vi "Is Sub-Path.vi"(9 "File Path 2":path, 11 "File Path":path) -> (0 "Relative File Path 2":path, 2 "File Path 2 a Sub-Path?":bool)   [LabVIEW 2010]
doc: "<B>Name:</B>\n Is Sub-Path.vi\n<B>References:</B>\n\n<B>Function Description:</B>\nThis VI returns TRUE if File Path 2 is a sub-path of File Path. It also returns the relative path from File Path to File Path 2.\n\nNote that a TRUE does not guarantee that the file path(s) exist or are valid.\n<B>Inputs:</B>\nFile path: Input path\nFile path 2: Input path for determining if if it is a sub-path of File Path.\n<B>Outputs:</B>\nFile Path 2 is a Sub Path?: Boolean result\nRelative file path 2: Relative path from File Path to File Path 2\n<B>Globals:</B>\n\n<B>TestStand Variables:</B>\n\n<B>User Guide:</B>\n\n<B>Control Usage Rules:</B>\n\n<B>VI Interaction:</B>\n\n<B>Occurences:</B>\n\n<B>Devices:</B>\n\n<B>Files:</B>\n\n<B>System Calls:</B>\n\n<B>Keywords:</B>\n\n<B>Initial Developer: Date:</B>\nMJShultz\n\nCurrent Revision: 26\nVSS Version: 3\nCopyright 2002 VI Engineering, Inc."
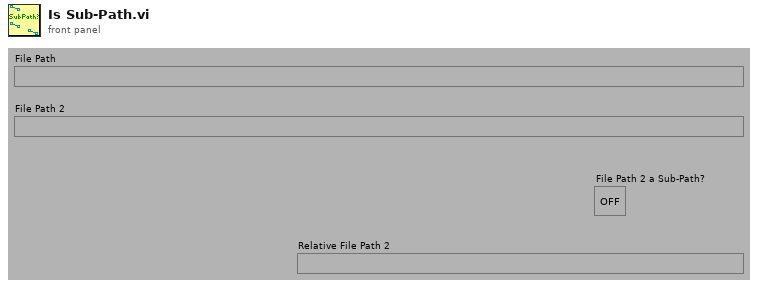
[diagram p1: front panel]
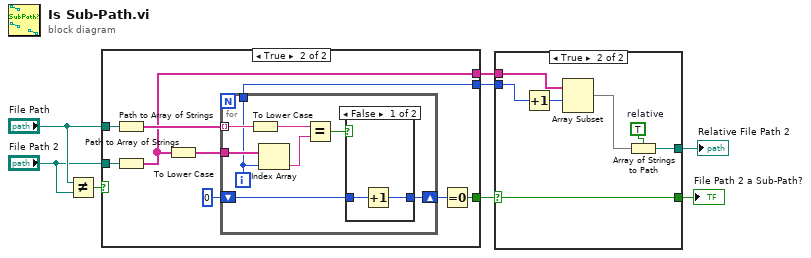
[diagram p0: block diagram]
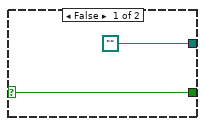
[diagram p2: hidden frame]
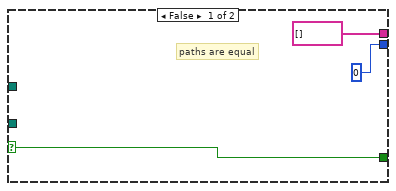
[diagram p3: hidden frame]
diagram:
  n1 = Not Equal?(x="File Path", y="File Path 2") -> (x != y?=w6:bool)
  n2 = case shown="True" w6 {
    selector: w6 -> [w11 _]
    tunnel: [w11 w17] -> w5
    tunnel: "File Path" -> [_ w16]
    tunnel: "File Path 2" -> [_ w15]
    tunnel: [0 w14] -> w3
    tunnel: [string[] [] ("array of strings") w13] -> w2
    frame False {
      # "paths are equal"
    }
    frame True {
      n3 = Path to Array of Strings(0:w16) -> (2:w20:string[])  [unwired: 1 out]
      n4 = Path to Array of Strings(0:w15) -> (2:w13:string[])  [unwired: 1 out]
      n5 = To Lower Case(string=w13) -> (all lower case string=w12:string[])
      n6 = for {
        tunnel: w20 -> [w26] mode=indexing
        tunnel: w12 -> [w28]
        shift-right: [w25] -> w18
        shift-left: 0 -> [w23]
        tunnel: [w22] -> w14
        i -> [w22]
        n7 = To Lower Case(string=w26) -> (all lower case string=w21:string)
        n8 = Index Array(array=w28, index=w22) -> (element=w27:string)
        n9 = Equal?(x=w21, y=w27) -> (x = y?=w24:bool)
        n10 = case shown="False" w24 {
          tunnel: [w29 w31] -> w25
          tunnel: w23 -> [w30 w31]
          frame False {
            n11 = Increment(x=w30) -> (x+1=w29:i32)
          }
          frame True {
          }
        }
      }
      n12 = Equal To 0?(x=w18) -> (x = 0?=w17:bool)
    }
  }
  n13 = case shown="True" w5 {
    selector: w5 -> [w33 w40]
    tunnel: [w33 w40] -> w4
    tunnel: w3 -> [_ w38]
    tunnel: w2 -> [_ w39]
    tunnel: [path "" w37] -> w1
    frame False {
    }
    frame True {
      w35 = TRUE  # relative
      n14 = Increment(x=w38) -> (x+1=w34:i32)
      n15 = Array Subset(array=w39, index=w34) -> (w36:string[])  [unwired: 1 in]
      n16 = Array of Strings to Path(0:w36, 1:w35) -> (2:w37:path)
    }
  }
  "File Path 2 a Sub-Path?" <- w4
  "Relative File Path 2" <- w1
